vi "First Law BAE7.vi"(2 "error in":errorcluster) -> (8 "error out":errorcluster)   [LabVIEW 2014]
doc: "First Law BAE7\n\nDisplays a dialouge until the ELVIS supplies 5 V through DC into AI3, or until they dismiss the prompt. In doing so, this serves to check if the First Law of Electronics is upheld, which inquires, if the machine is turned on.\n\nBeverly Abadines\nPHY 350\nE7"
panel:
  # "Beverly Abadines\nPhys 350\nE7"
  # "First Law BAE7"
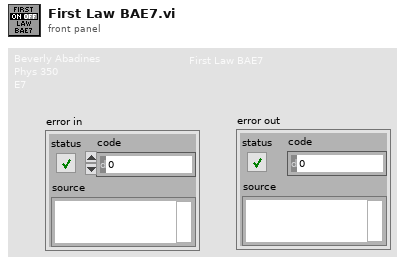
[diagram p1: front panel]
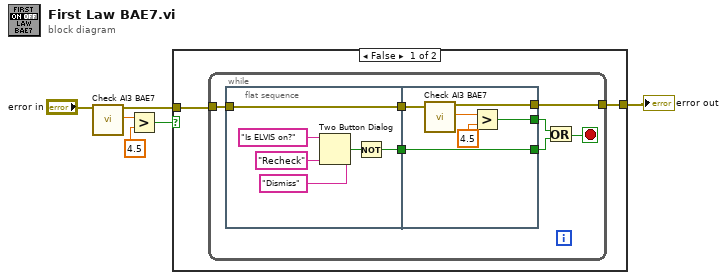
[diagram p0: block diagram]
diagram:
  n1 = call "Check AI3 BAE7.vi"("error in"="error in") -> ("error out"=w4:errorcluster, "voltage out"=w2:dbl)  [unwired: 17 in]
  n2 = Greater?(x=w2, y=4.5) -> (0:w1:bool)
  n3 = case shown="False" w1 {
    tunnel: [w7 w28] -> w6
    tunnel: w4 -> [w8 w28]
    frame False {
      n4 = while {
        tunnel: w8 -> [w12]
        tunnel: [w10] -> w7
        stop <- w15 stop-if-true
        n5 = flat-sequence {
          tunnel: [w18] -> w13
          tunnel: w12 -> [w16]
          tunnel: [w16] -> w11
          tunnel: [w27] -> w14
          tunnel: w13 -> [w27]
          tunnel: w11 -> [w25]
          tunnel: [w24] -> w10
          tunnel: [w22] -> w9
          frame #0 {
            n6 = Two Button Dialog(message="Is ELVIS on?", 1:"Dismiss" ("F button name (\"Cancel\")"), 2:"Recheck" ("T button name (\"OK\")")) -> (T button?=w21:bool)
            n7 = Not(x=w21) -> (.not. x?=w18:bool)
          }
          frame #1 {
            n8 = call "Check AI3 BAE7.vi"("error in"=w25) -> ("error out"=w24:errorcluster, "voltage out"=w26:dbl)  [unwired: 17 in]
            n9 = Greater?(x=w26, y=4.5) -> (0:w22:bool)
          }
        }
        n10 = Or(x=w9, y=w14) -> (x .or. y?=w15:bool)
      }
    }
    frame True {
    }
  }
  "error out" <- w6
